vi "ADC_Triggered.vi"(8 "error in (no error)":errorcluster) -> (0 "error out":errorcluster, 3 "function return":i16)   [LabVIEW 2013, in "MeasurmentRoutines.lvlib"]
doc: "Description: This routine reads the trigger status from the hardware. The returned value indicates which trigger source caused the trigger, this value is different for various instruments.\nInput: -\nOutput: Return value HS4 / HS4 DIFF other instruments\n0 not triggered not triggered\n1 Ch1 Ch1\n2 Ch2 Ch2\n4 Ch3 External\n8 Ch4 -\n16 External -\nRemark: Return value can be a combination of indicated values.\n\nFunction prototype: word ADC_Triggered( void )\n\n\n\nshort int ADC_Triggered ( void );"
uses:
  MeasurmentRoutines.lvlib
  hs3.dll
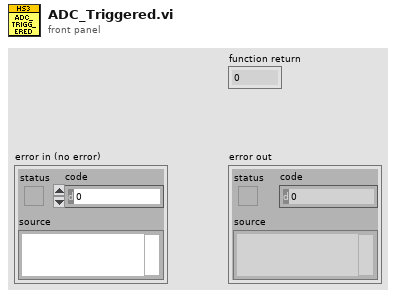
[diagram p1: front panel]
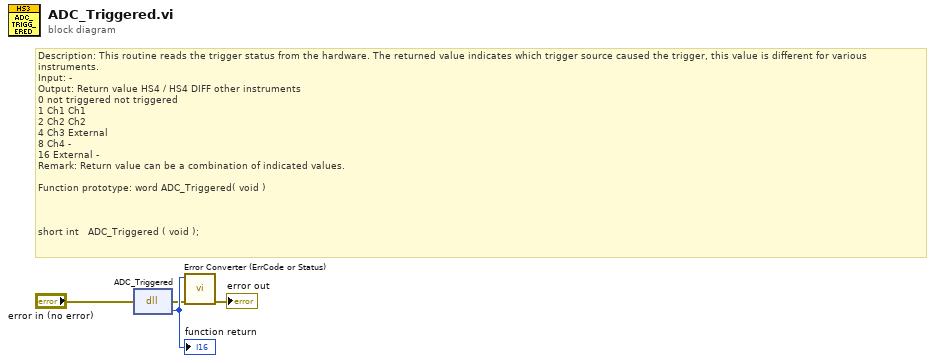
[diagram p0: block diagram]
diagram:
  # "Description: This routine reads the trigger status from the hardware. The returned value indicates which trigger source caused the trigger, this value is different for various instruments.\nInput: -\nOutput: Return value HS4 / HS4 DIFF other instruments\n0 not triggered not triggered\n1 Ch1 Ch1\n2 Ch2 Ch2\n4 Ch3 External\n8 Ch4 -\n16 External -\nRemark: Return value can be a combination of indicated values.\n\nFunction prototype: word ADC_Triggered( void )\n\n\n\nshort int \t\tADC_Triggered\t( void );"
  n1 = dll-call lib="C:/Documents and Settings/admin/Pulpit/HS3 LabViewLib/HS3_WRAPPER/hs3.*" fn="ADC_Triggered"(error in="error in (no error)") -> (error out=w2:errorcluster, w4:i16)  [unwired: 2 in, 1 out]
  "function return" <- w4
  n2 = call "Error Converter (ErrCode or Status).vi"("error in (no error)"=w2, "error code"=w4) -> ("error out"=→"error out":errorcluster)  [unwired: 9 in]
